vi "OE1022D_Configure Input Filter.vi"(7 "OE1022D_Configure Input Filter":T1={"Input Source"=0, "Input Shield Grounding "=0, "Input Coupling "=0, "Input Notch Filter "=0, "Channel"=1} {"Channel" items=["A"=1, "B"=2]; "Input Notch Filter" items=["None"=0, "50Hz"=1, "100Hz"=3, "Both"=2]; "Input Coupling" items=["AC", "DC"]; "Input Shield Grounding" items=["Float", "Ground"]; "Input Source" items=["A", "B", "I-1M", "I-100M"]}, 8 "Error in (no error)":errorcluster caption="error out（no error）", 9 "Remote Mode":u16(ring) items=["USB", "RS232", "GPIB"], 11 "VISA resource name":refnum<visa-resource-name>) -> (0 "Error out":errorcluster caption="error out", 1 "Output String":string, 3 "VISA resource  out":refnum<visa-resource-name>)   [LabVIEW 2011]
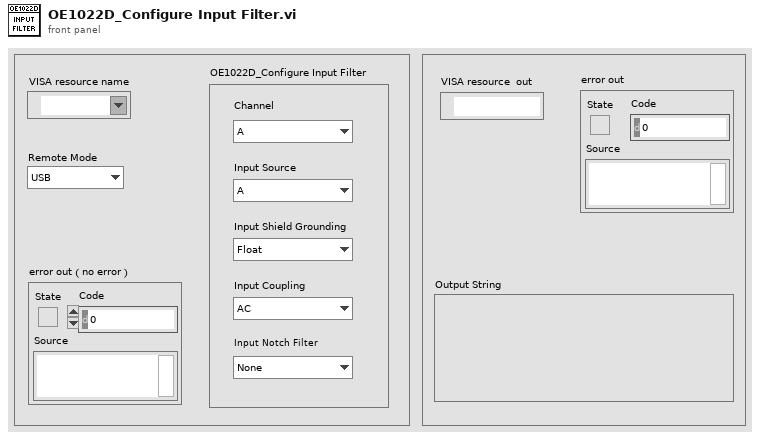
[diagram p1: front panel]
types:
  T1 = cluster{"Input Source":u16, "Input Shield Grounding ":u16, "Input Coupling ":u16, "Input Notch Filter ":u16, "Channel":u16}
  T2 = enum16{"ISRC", "IGND", "ICPL", "ILIN", "PHAS", "FMOD", "RSLP", "FREQ", "SWPT", "SLLM", "SULM", "SSLL", "SSLG", "STLM", "SWRM", "IRNG", "SENS", "RMOD", "OFLT", "OFSL", "SYNC", "DMOD", "HARM", "DARB", "SWVT", "SLVL", "SVLL", "SVUL", "SVSL", "SVSG", "SVTM", "SVRM", "RALL", "SNAP", "OUTP", "OAUX", "COUT", "CAUX", "COFP", "CEXP", "FPOP", "OEXP", "*IDN", "*RST", "OVLD", "INOV", "GNOV", "*PLL", "SSET", "RSET", "AGAN", "APHS", "ARSV", "ASCL", "EQCD", "EQCS", "SPED", "SRAT", "SLEN", "SSLE", "STRG", "SPRM", "STRD", "PAUS", "REST", "SPTS", "TRCA", "TEMP", "RSTU", "IHNZ", "DEQU", "SADD", "ARNG", "CSPE", "ISRCD", "IGNDD", "ICPLD", "ILIND", "PHASD", "FMODD", "RSLPD", "FREQD", "SWPTD", "SLLMD", "SULMD", "SSLLD", "SSLGD", "STLMD", "SWRMD", "SENSD", "RMODD", "OFLTD", "OFSLD", "SYNCD", "HARMD", "EQCDD", "EQCSD", "SNAPD", "OUTPD", "SWVTD", "SLVLD", "SVLLD", "SVULD", "SVSLD", "SVSGD", "SVTMD", "SVRMD", "SVDCD", "ARSVD", "AGAND", "APHSD", "ASCLD", "FPOPD", "CAUXD", "OEXPD", "SPEDD", "SRATD", "SLEND", "SSLED", "STRGD", "SPRMD", "STRDD", "PAUSD", "RESTD", "SPTSD", "TRCAD", "*IDND", "*RSTD", "INOVD", "GNOVD", "*PLLD", "SSETD", "RSETD"}
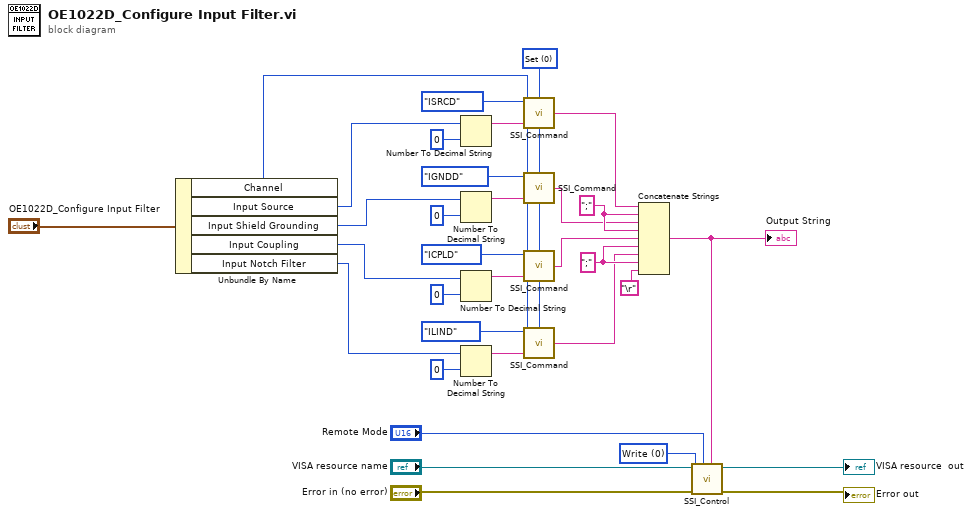
[diagram p0: block diagram]
diagram:
  w20 = ";" ("字符串")
  w19 = ";" ("字符串")
  w21 = u16 0 items=["Set", "Query"] ("Opera")
  w32 = u16 0 items=["Write", "Read"] ("Control")
  n1 = Unbundle By Name("OE1022D_Configure Input Filter") -> ("Channel"=w1:u16, "Input Source"=w22:u16, "Input Shield Grounding"=w23:u16, "Input Coupling"=w24:u16, "Input Notch Filter"=w25:u16)
  n2 = Number To Decimal String(number=w22, width (-)=i16 0 ("精度(6)")) -> (decimal integer string=w4:string)
  n3 = Number To Decimal String(number=w23, width (-)=i16 0 ("精度(6)")) -> (decimal integer string=w7:string)
  n4 = Number To Decimal String(number=w24, width (-)=i16 0 ("精度(6)")) -> (decimal integer string=w12:string)
  n5 = Number To Decimal String(number=w25, width (-)=i16 0 ("精度(6)")) -> (decimal integer string=w15:string)
  n6 = call "SSI_Command.vi"("Opera"=w21, "Paramter"=w4, "channel"=w1, "Command Type"=T2."ISRCD") -> ("Output string"=w9:string)
  n7 = call "SSI_Command.vi"("Opera"=w21, "Paramter"=w7, "channel"=w1, "Command Type"=T2."IGNDD") -> ("Output string"=w10:string)
  n8 = call "SSI_Command.vi"("Opera"=w21, "Paramter"=w12, "channel"=w1, "Command Type"=T2."ICPLD") -> ("Output string"=w18:string)
  n9 = call "SSI_Command.vi"("Opera"=w21, "Paramter"=w15, "channel"=w1, "Command Type"=T2."ILIND") -> ("Output string"=w17:string)
  n10 = Concatenate Strings(w9, w19, w10, w19, w18, w20, w17, w20, "\r") -> (w2:string)
  "Output String" <- w2
  n11 = call "SSI_Control.vi"("Write Buffer"=w2, "Remote Mode"="Remote Mode", "Error in (no error)"="Error in (no error)", "Control"=w32, "VISA resource name"="VISA resource name") -> ("Error out"=→"Error out":errorcluster, "VISA resource  out"=→"VISA resource  out":refnum<visa-resource-name>)  [unwired: 3 in, 2 out]
